vi "Reset.vi"(8 "error in (no error)":errorcluster, 11 "3446X in":refnum<class "3446X.lvclass">) -> (0 "error out":errorcluster, 3 "3446X out":refnum<class "3446X.lvclass">)   [LabVIEW 2018, in "3446X.lvlib" / "3446X.lvclass"]
uses:
  3446X.lvclass
  3446X.lvclass/3446X.ctl
  <instrlib>/Agilent 3446X Series/Agilent 3446X Series.lvlib
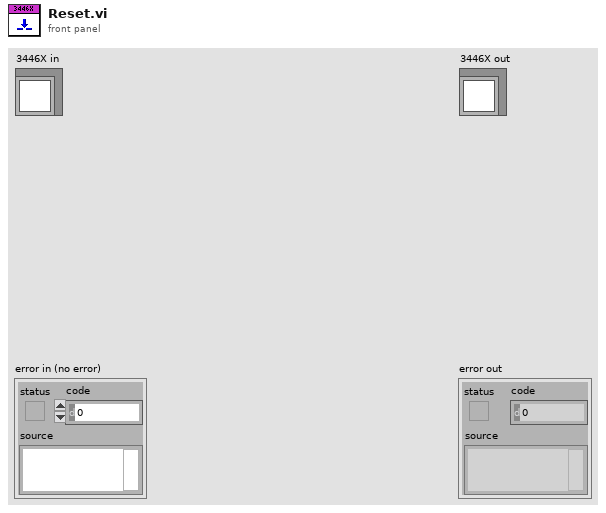
[diagram p1: front panel]
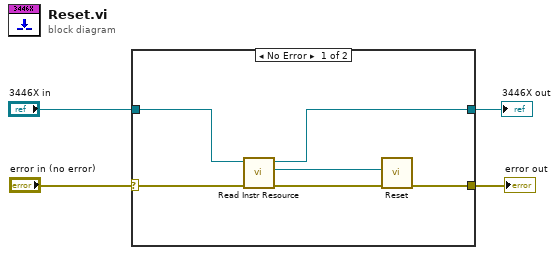
[diagram p0: block diagram]
diagram:
  n1 = case shown="No Error" "error in (no error)" {
    selector: "error in (no error)" -> [w10 w11]
    tunnel: [w8 w11] -> w3
    tunnel: "3446X in" -> [w7 w12]
    tunnel: [w6 w12] -> w1
    frame No Error {
      n2 = call "Read Instr Resource.vi"("error in (no error)"=w10, "3446X in"=w7) -> ("error out"=w9:errorcluster, "Instr Resource"=w5:refnum<visa-resource-name>, "3446X out"=w6:refnum<class "3446X.lvclass">)  [unwired: 7 in]
      n3 = call <instrlib>:"Reset.vi"("error in (no error)"=w9, "VISA resource name"=w5) -> ("error out"=w8:errorcluster)  [unwired: 8 in, 1 out]
    }
    frame Error {
    }
  }
  "error out" <- w3
  "3446X out" <- w1
